vi "Get GUI reference.vi"(8 "error in (no error)":errorcluster, 11 "Optimiser SBlock in":refnum<class "Optimiser SBlock.lvclass">) -> (0 "error out":errorcluster, 2 "reference out":refnum<vi>, 3 "Optimiser SBlock out":refnum<class "Optimiser SBlock.lvclass">)   [LabVIEW 2020, in "TALOS.lvlib" / "Run Utilities.lvlib" / "Optimiser SBlock.lvclass"]
doc: "Create a GUI element for this SBlock"
uses:
  Optimiser SBlock.lvclass
  Optimiser Cell/Optimise parameter - numeric.ctl
  Optimiser Cell/Optimise parameter - string.ctl
  Optimiser Cell/Optimisation observable.ctl
  Optimiser Cell/Optimiser Cell.lvclass
panel:
  out "Observables":T1[](array[typedef]) {"Weight" min=0.0 max=1.0}
  out "Parameters - String":T2[](array[typedef])
  out "Parameters - Numertic":T3[](array[typedef])
  out "Explor.\nRUNs":u32
  out "Strategy":string
  out "Common Parameters":string[][](array[string])
  out "Kasli":string
  out "Number of repetitions":u16=1 min=1
  out "Script name":string
  # "s"
  # "Observables"
  # "Weight"
  # "Parameters- String"
  # "Start value"
  # "List of values"
  # "Start value"
  # "Parameters - Numeric"
  # "From"
  # "To"
  # "dtype"
  # "Parameter Name"
  # "Parameter Value"
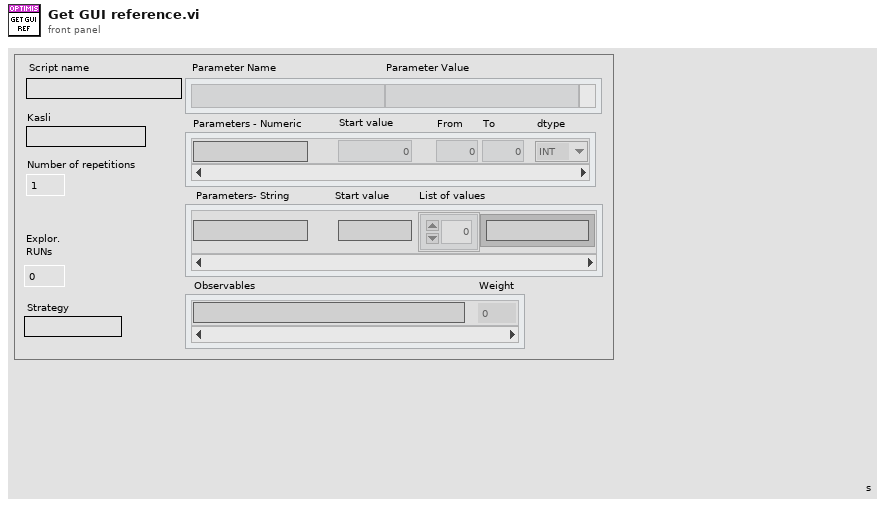
[diagram p1: front panel]
types:
  T1 = typedef "TALOS.lvlib/Run Utilities.lvlib/Optimiser Cell.lvclass/Optimisation observable.ctl" = cluster{"Name":string, "Weight":dbl}
  T2 = typedef "TALOS.lvlib/Run Utilities.lvlib/Optimiser Cell.lvclass/Optimise parameter - string.ctl" = cluster{"Name":string, "Start value":string, "Options":string[]}
  T3 = typedef "TALOS.lvlib/Run Utilities.lvlib/Optimiser Cell.lvclass/Optimise parameter - numeric.ctl" = cluster{"Name":string, "Start value":dbl, "From":dbl, "To":dbl, "dtype":enum16{"INT", "DBL"}}
  T4 = typedef "TALOS.lvlib/Run Utilities.lvlib/Optimiser Cell.lvclass/Optimisation Strategy.ctl" = enum16{"Maximize", "Minimize", "Value"}
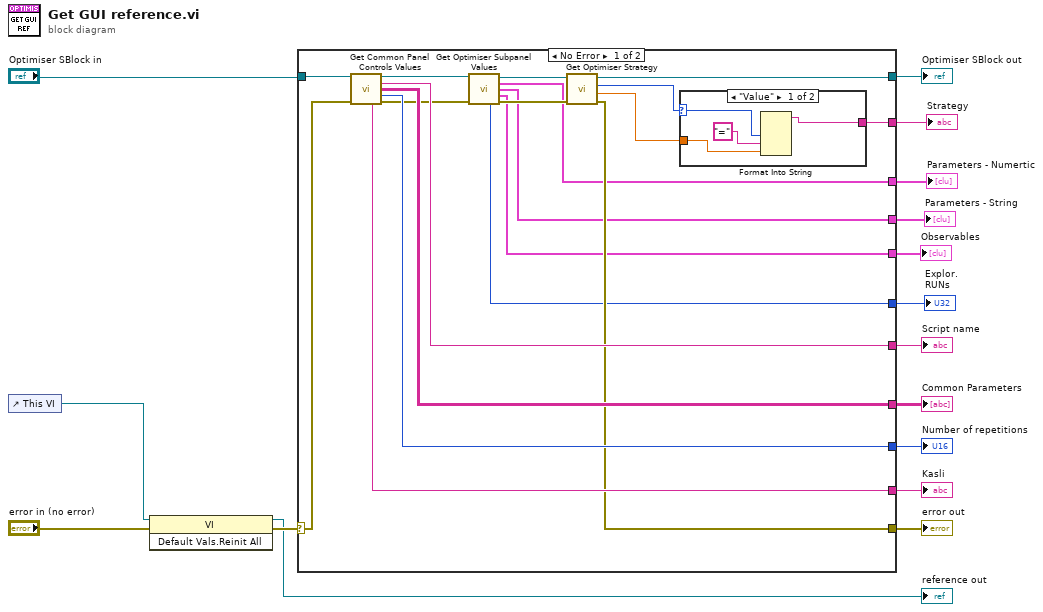
[diagram p0: block diagram]
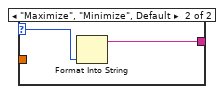
[diagram p2: hidden frame]
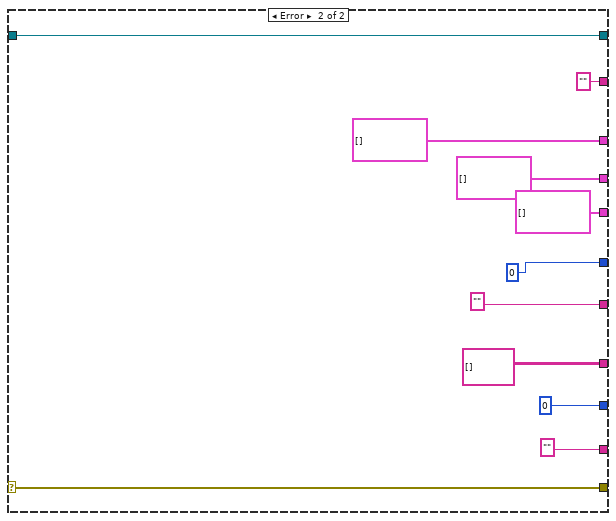
[diagram p3: hidden frame]
diagram:
  n1 = control-ref of="This VI"() -> (w15:refnum<vi>)
  n2 = invoke class="VI" method="Default Vals.Reinit All"(reference=w15, error in="error in (no error)") -> (reference out=→"reference out":refnum<vi>, error out=w13:errorcluster)  [unwired: 1 in, 1 out]
  n3 = case shown="No Error" w13 {
    selector: w13 -> [w34 w52]
    tunnel: [w24 w52] -> w11
    tunnel: [w25 w51] -> w10
    tunnel: "Optimiser SBlock in" -> [w35 w51]
    tunnel: [w33 "" ("Kasli Name")] -> w9
    tunnel: [w32 u16 0 ("Number of repetitions")] -> w8
    tunnel: [w31 string[][] [] ("Common Parameters")] -> w7
    tunnel: [w30 "" ("Script Name")] -> w6
    tunnel: [w23 u32 0 ("No. of steps")] -> w5
    tunnel: [w22 T1[] [] ("Observables")] -> w4
    tunnel: [w21 T2[] [] ("Parameters - String")] -> w3
    tunnel: [w20 T3[] [] ("Parameters - Numeric")] -> w2
    tunnel: [w17 ""] -> w1
    frame No Error {
      n4 = call-dynamic "Get Common Panel Controls Values.vi"("Schedule Block in"=w35, "error in (no error)"=w34) -> ("Schedule Block out"=w29:refnum<class "Optimiser SBlock.lvclass">, "Script Name"=w30:string, "Common Parameters"=w31:string[][], "Number of repetitions"=w32:u16, "FPGA Name"=w33:string, "error out"=w28:errorcluster)  [unwired: 7 in, 1 out]
      n5 = call "Get Optimiser Subpanel Values.vi"("Optimiser SBlock in"=w29, "error in (no error)"=w28) -> ("Optimiser SBlock out"=w26:refnum<class "Optimiser SBlock.lvclass">, "Parameters - Numeric"=w20:T3[], "Parameters - String"=w21:T2[], "Observables"=w22:T1[], "Number of Exploration Runs"=w23:i32, "error out"=w27:errorcluster)  [unwired: 8 in]
      n6 = call-dynamic "Get Optimiser Strategy.vi"("error in (no error)"=w27, "Optimiser SBlock in"=w26) -> ("error out"=w24:errorcluster, "Value"=w18:dbl, "Optimisation Strategy"=w19:T4, "Optimiser SBlock out"=w25:refnum<class "Optimiser SBlock.lvclass">)  [unwired: 6 in]
      n7 = case shown="\"Value\"" w19 {
        selector: w19 -> [w39 w41]
        tunnel: w18 -> [w38 _]
        tunnel: [w36 w40] -> w17
        frame "Value" {
          n8 = Format Into String(w39, "=", w38) -> (resulting string=w36:string)  [unwired: 3 in, 1 out]
        }
        frame "Maximize", "Minimize", Default {
          n9 = Format Into String(w41) -> (resulting string=w40:string)  [unwired: 3 in, 1 out]
        }
      }
    }
    frame Error {
    }
  }
  "error out" <- w11
  "Optimiser SBlock out" <- w10
  "Script name" <- w6
  "Number of repetitions" <- w8
  "Common Parameters" <- w7
  "Kasli" <- w9
  "Explor.\nRUNs" <- w5
  "Parameters - Numertic" <- w2
  "Parameters - String" <- w3
  "Observables" <- w4
  "Strategy" <- w1
